vi "Configure Multi Eval Meas Modulation EVM Vs Symbol Scope.vi"(7 "Window Position (Low)":i32(ring) items=["Low", "High"], 8 "error in (no error)":errorcluster, 9 "Symbol (0)":i32, 10 "Instance (1)":T1=1, 11 "VISA resource name":refnum<visa-resource-name>) -> (0 "error out":errorcluster, 3 "VISA resource name out":refnum<visa-resource-name>)   [LabVIEW 2020, in "Rohde&Schwarz CMXP NR FR2 Measurement.lvlib"]
doc: "Configures the scope of the EVM vs modulation symbol results.\n\nAttribute:\nRSCMXPNRFR2M_ATTR_MULTI_EVAL_MEASUREMENT_MODULATION_EVM_VS_SYMBOL_SCOPE\n\nRemote-control command:\nCONFigure:NRMMw:MEAS<i>:MEValuation:MODulation:EVMSymbol"
uses:
  <instrlib>/Rohde&Schwarz CMXP NR FR2 Measurement/Rohde&Schwarz CMXP NR FR2 Measurement.lvlib
  <instrlib>/Rohde&Schwarz CMXP NR FR2 Measurement/Private/_Instance.ctl
  <instrlib>/Rohde&Schwarz CMXP NR FR2 Measurement/Private/rsidr_core.llb/rsidr_core.lvlib
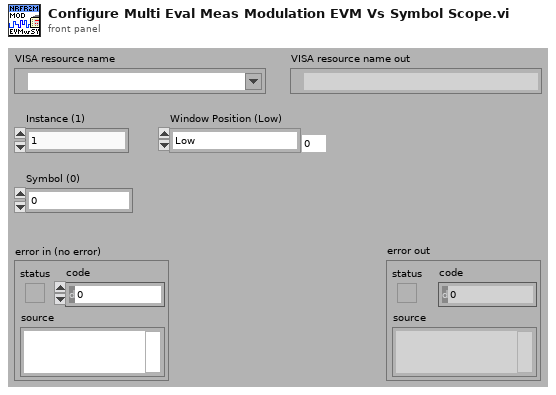
[diagram p1: front panel]
types:
  T1 = typedef "Rohde&Schwarz CMXP NR FR2 Measurement.lvlib/_Instance.ctl" = i32
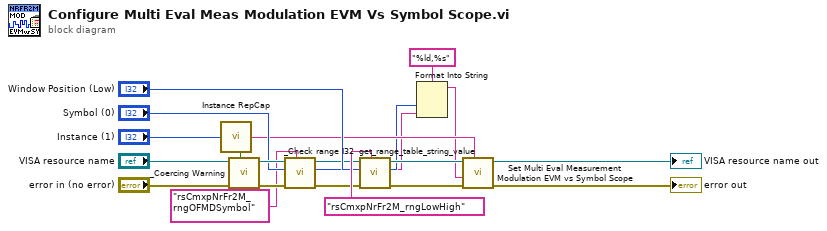
[diagram p0: block diagram]
diagram:
  n1 = call <instrlib>:"Instance RepCap.vi"("Instance In"="Instance (1)") -> ("In Range?"=w19:bool, "RepCap Identifier Out"=w9:string)  [unwired: 1 in]
  n2 = call <instrlib>:"_Coercing Warning.vi"("In Range?"=w19, "error in (no error)"="error in (no error)", "VISA resource name"="VISA resource name") -> ("error out"=w18:errorcluster, "VISA resource name out"=w17:refnum<visa-resource-name>)  [unwired: 7 in]
  n3 = call <instrlib>:"_Check range I32.vi"("Range Table Identifier"="rsCmxpNrFr2M_rngOFMDSymbol", "error in (no error)"=w18, "I32 Value In"="Symbol (0)", "VISA resource name"=w17) -> ("error out"=w11:errorcluster, "I32 Value Out"=w4:i32, "VISA resource name out"=w12:refnum<visa-resource-name>)  [unwired: 5 in]
  n4 = call <instrlib>:"get_range_table_string_value.vi"("Range Table ID in"="rsCmxpNrFr2M_rngLowHigh", "error in"=w11, "I32 input"="Window Position (Low)", "VISA resource name"=w12) -> ("error out"=w7:errorcluster, "String Value out"=w3:string, "VISA resource name out"=w8:refnum<visa-resource-name>)  [unwired: 5 in]
  n5 = Format Into String(format string="%ld,%s", w4, w3) -> (resulting string=w1:string)  [unwired: 2 in, 1 out]
  n6 = call "Set Multi Eval Measurement Modulation EVM vs Symbol Scope"("Repeated Capabilities"=w9, "error in (no error)"=w7, "Multi Eval Measurement Modulation EVM vs Symbol Scope ()"=w1, "instrument handle"=w8) -> ("error out"=→"error out":errorcluster, "instrument handle out"=→"VISA resource name out":refnum<visa-resource-name>)  [unwired: 6 in]
